vi "ai_oneshot_ext_trig_in.vi"() -> ()   [LabVIEW 2020]
uses:
  <vilib>/Platform/TimedLoop/XDataNode/timing_clust.ctl
  <vilib>/Platform/TimedLoop/XDataNode/nitl_modes.ctl
  <vilib>/Platform/TimedLoop/XDataNode/wakeup.ctl
  <vilib>/platform/TimedLoop/XDataNode/XDataNode.xnode
  <vilib>/Platform/TimedLoop/XDataNode/XDNodeRunTimeDep.lvlib
panel:
  out "loop":i32
  in  "stop":bool
  in  "AiOneShotPoints":u32=500
  out "error out":errorcluster caption="错误输出"
  out "AiFifoResidual":i32
  out "波形图":sgl[][](graph)=[[1.0535451, 1.0535451, 1.0633912, 1.0584682, 1.0535451, 1.0535451, 1.0535451, 1.0535451, 1.0535451, 1.0535451, 1.0535451, 1.0486219, 1.0535451, 1.0486219, 1.0535451, 1.0535451, 1.0535451, 1.0535451, 1.0535451, 1.0535451, 1.0535451, 1.0535451, 1.0486219, 1.0535451, 1.0535451, 1.0535451, 1.0535451, 1.0535451, 1.0535451, 1.0535451, 1.0535451, 1.0486219, 1.0535451, 1.0535451, 1.0535451, 1.0535451, 1.0535451, 1.0535451, 1.0535451, 1.0584682, 1.0535451, 1.0535451, 1.0535451, 1.0535451, 1.0535451, 1.0535451, 1.0535451, 1.0535451, 1.0584682, 1.0535451, 1.0535451, 1.0535451, 1.0535451, 1.0535451, 1.0535451, 1.0535451, 1.0584682, 1.0584682, 1.0535451, 1.0584682, 1.0584682, 1.0584682, 1.0535451, 1.0535451, 1.0584682, 1.0535451, 1.0584682, 1.0535451, 1.0535451, 1.0535451, 1.0584682, 1.0535451, 1.0535451, 1.0535451, 1.0535451, 1.0584682, 1.0535451, 1.0535451, 1.0584682, 1.0535451, 1.0535451, 1.0535451, 1.0535451, 1.0535451, 1.0584682, 1.0535451, 1.0535451, 1.0535451, 1.0535451, 1.0535451, 1.0535451, 1.0535451, 1.0535451, 1.0535451, 1.0535451, 1.0535451, 1.0535451, 1.0535451, 1.0535451, 1.0535451, 1.0535451, 1.0535451, 1.0535451, 1.0486219, 1.0535451, 1.0535451, 1.0535451, 1.0535451, 1.0535451, 1.0535451, 1.0535451, 1.0535451, 1.0535451, 1.0535451, 1.0535451, 1.0535451, 1.0535451, 1.0535451, 1.0535451, 1.0535451, 1.0535451, 1.0535451, 1.0535451, 1.0535451, 1.0535451, 1.0535451, 1.0535451, 1.0535451, 1.0535451, 1.0535451, 1.0535451, 1.0535451, 1.0535451, 1.0584682, 1.0584682, 1.0584682, 1.0535451, 1.0584682, 1.0584682, 1.0584682, 1.0584682, 1.0633912, 1.0633912, 1.0633912, 1.0633912, 1.0633912, 1.0633912, 1.0633912, 1.0584682, 1.0633912, 1.0584682, 1.0584682, 1.0584682, 1.0584682, 1.0584682, 1.0584682, 1.0633912, 1.0584682, 1.0584682, 1.0584682, 1.0633912, 1.0633912, 1.0584682, 1.0584682, 1.0584682, 1.0633912, 1.0584682, 1.0584682, 1.0584682, 1.0584682, 1.0584682, 1.0584682, 1.0584682, 1.0584682, 1.0584682, 1.0535451, 1.0535451, 1.0535451, 1.0535451, 1.0535451, 1.0535451, 1.0535451, 1.0535451, 1.0535451, 1.0486219, 1.0535451, 1.0535451, 1.0535451, 1.0535451, 1.0535451, 1.0535451, 1.0535451, 1.0535451, 1.0535451, 1.0535451, 1.0535451, 1.0535451, 1.0535451, 1.0535451, 1.0535451, 1.0535451, 1.0535451, 1.0535451, 1.0535451, 1.0535451, 1.0535451, 1.0535451, 1.0535451, 1.0535451, 1.0535451, 1.0584682, 1.0535451, 1.0535451, 1.0584682, 1.0584682, 1.0584682, 1.0584682, 1.0584682, 1.0584682, 1.0584682, 1.0535451, 1.0584682, 1.0584682, 1.0584682, 1.0584682, 1.0584682, 1.0584682, 1.0584682, 1.0584682, 1.0535451, 1.0584682, 1.0584682, 1.0584682, 1.0584682, 1.0584682, 1.0584682, 1.0584682, 1.0633912, 1.0584682, 1.0584682, 1.0584682, 1.0584682, 1.0584682, 1.0584682, 1.0584682, 1.0584682, 1.0584682, 1.0535451, 1.0535451, 1.0584682, 1.0584682, 1.0535451, 1.0535451, 1.0535451, 1.0535451, 1.0535451, 1.0486219, 1.0535451, 1.0535451, 1.0535451, 1.0535451, 1.0535451, 1.0535451, 1.0535451, 1.0535451, 1.0486219, 1.0535451, 1.0535451, 1.0535451, 1.0486219, 1.0486219, 1.0486219, 1.0486219, 1.0486219, 1.0486219, 1.0486219, 1.0486219, 1.0486219, 1.0486219, 1.0486219, 1.0486219, 1.0486219, 1.0486219, 1.0486219, 1.0486219, 1.0486219, 1.0486219, 1.0486219, 1.0486219, 1.0486219, 1.0486219, 1.0535451, 1.0486219, 1.0486219, 1.0486219, 1.0486219, 1.0486219, 1.0486219, 1.0486219, 1.0486219, 1.0486219, 1.0486219, 1.0486219, 1.0486219, 1.0535451, 1.0486219, 1.0486219, 1.0535451, 1.0535451, 1.0535451, 1.0486219, 1.0535451, 1.0535451, 1.0535451, 1.0535451, 1.0535451, 1.0535451, 1.0584682, 1.0584682, 1.0584682, 1.0584682, 1.0584682, 1.0633912, 1.0633912, 1.0584682, 1.0633912, 1.0633912, 1.0633912, 1.0633912, 1.0633912, 1.0633912, 1.0633912, 1.0633912, 1.0633912, 1.0633912, 1.0683143, 1.0683143, 1.0633912, 1.0633912, 1.0633912, 1.0683143, 1.0633912, 1.0683143, 1.0683143, 1.0683143, 1.0683143, 1.0633912, 1.0683143, 1.0683143, 1.0683143, 1.0683143, 1.0683143, 1.0683143, 1.0633912, 1.0683143, 1.0633912, 1.0633912, 1.0633912, 1.0633912, 1.0633912, 1.0633912, 1.0633912, 1.0633912, 1.0633912, 1.0584682, 1.0633912, 1.0584682, 1.0584682, 1.0584682, 1.0584682, 1.0584682, 1.0584682, 1.0584682, 1.0535451, 1.0584682, 1.0584682, 1.0584682, 1.0584682, 1.0584682, 1.0584682, 1.0535451, 1.0535451, 1.0486219, 1.0535451, 1.0535451, 1.0535451, 1.0535451, 1.0535451, 1.0486219, 1.0486219, 1.0486219, 1.0486219, 1.0486219, 1.0486219, 1.0486219, 1.0486219, 1.0486219, 1.0486219, 1.0486219, 1.0486219, 1.0436989, 1.0486219, 1.0486219, 1.0486219, 1.0486219, 1.0486219, 1.0486219, 1.0486219, 1.0486219, 1.0436989, 1.0486219, 1.0486219, 1.0486219, 1.0486219, 1.0486219, 1.0486219, 1.0486219, 1.0486219, 1.0436989, 1.0486219, 1.0535451, 1.0486219, 1.0486219, 1.0535451, 1.0486219, 1.0535451, 1.0535451, 1.0486219, 1.0535451, 1.0535451, 1.0535451, 1.0535451, 1.0535451, 1.0535451, 1.0535451, 1.0535451, 1.0486219, 1.0535451, 1.0535451, 1.0535451, 1.0535451, 1.0535451, 1.0535451, 1.0535451, 1.0535451, 1.0486219, 1.0535451, 1.0535451, 1.0535451, 1.0535451, 1.0535451, 1.0535451, 1.0535451, 1.0535451, 1.0535451, 1.0535451, 1.0535451, 1.0535451, 1.0535451, 1.0535451, 1.0535451, 1.0535451, 1.0584682, 1.0535451, 1.0584682, 1.0584682, 1.0584682, 1.0584682, 1.0584682, 1.0584682, 1.0584682, 1.0584682, 1.0584682, 1.0633912, 1.0633912, 1.0633912, 1.0633912, 1.0633912, 1.0633912, 1.0633912, 1.0633912, 1.0584682, 1.0633912, 1.0633912, 1.0633912, 1.0633912, 1.0633912, 1.0633912, 1.0633912, 1.0633912, 1.0633912, 1.0633912, 1.0633912, 1.0683143, 1.0633912, 1.0633912, 1.0683143, 1.0633912, 1.0683143, 1.0633912, 1.0633912, 1.0683143, 1.0683143, 1.0633912, 1.0633912, 1.0633912, 1.0633912, 1.0584682, 1.0535451, 1.0486219, 1.0436989, 1.0436989, 1.0387758, 1.0338527, 1.0338527, 1.0338527, 1.0338527, 1.0240065, 1.0289296, 1.0289296, 1.0289296, 1.0289296, 1.0289296, 1.0289296, 1.0289296, 1.0289296, 1.0240065, 1.0338527, 1.0338527, 1.0338527, 1.0338527, 1.0338527, 1.0387758, 1.0387758, 1.0387758, 1.0387758, 1.0436989, 1.0436989, 1.0436989, 1.0436989, 1.0486219, 1.0486219, 1.0486219, 1.0535451, 1.0535451, 1.0535451, 1.0535451, 1.0584682, 1.0584682, 1.0584682], [1.0581981, 1.0581981, 1.0581981, 1.0631206, 1.0581981, 1.0581981, 1.0581981, 1.0581981, 1.0581981, 1.0581981, 1.0581981, 1.0532755, 1.0581981, 1.0581981, 1.0581981, 1.0581981, 1.0581981, 1.0581981, 1.0581981, 1.0631206, 1.0581981, 1.0631206, 1.0631206, 1.0631206, 1.0631206, 1.0631206, 1.0631206, 1.0680432, 1.0631206, 1.0631206, 1.0680432, 1.0631206, 1.0680432, 1.0631206, 1.0631206, 1.0631206, 1.0631206, 1.0631206, 1.0581981, 1.0631206, 1.0631206, 1.0631206, 1.0581981, 1.0581981, 1.0581981, 1.0581981, 1.0581981, 1.0581981, 1.0581981, 1.0581981, 1.0581981, 1.0532755, 1.0532755, 1.0532755, 1.0532755, 1.0532755, 1.0483528, 1.0532755, 1.0532755, 1.0532755, 1.0532755, 1.0532755, 1.0483528, 1.0532755, 1.0483528, 1.0434302, 1.0483528, 1.0483528, 1.0483528, 1.0483528, 1.0483528, 1.0483528, 1.0483528, 1.0483528, 1.0434302, 1.0483528, 1.0434302, 1.0483528, 1.0434302, 1.0434302, 1.0434302, 1.0434302, 1.0483528, 1.0434302, 1.0483528, 1.0483528, 1.0483528, 1.0434302, 1.0483528, 1.0483528, 1.0483528, 1.0483528, 1.0434302, 1.0483528, 1.0483528, 1.0532755, 1.0483528, 1.0483528, 1.0483528, 1.0483528, 1.0483528, 1.0483528, 1.0532755, 1.0532755, 1.0532755, 1.0532755, 1.0532755, 1.0532755, 1.0532755, 1.0532755, 1.0532755, 1.0581981, 1.0581981, 1.0581981, 1.0581981, 1.0581981, 1.0581981, 1.0631206, 1.0631206, 1.0581981, 1.0631206, 1.0631206, 1.0631206, 1.0631206, 1.0680432, 1.0680432, 1.0680432, 1.0680432, 1.0631206, 1.0680432, 1.0631206, 1.0631206, 1.0631206, 1.0631206, 1.0631206, 1.0631206, 1.0581981, 1.0581981, 1.0631206, 1.0581981, 1.0631206, 1.0581981, 1.0581981, 1.0581981, 1.0581981, 1.0581981, 1.0532755, 1.0581981, 1.0532755, 1.0581981, 1.0532755, 1.0532755, 1.0532755, 1.0532755, 1.0532755, 1.0483528, 1.0483528, 1.0483528, 1.0483528, 1.0483528, 1.0483528, 1.0483528, 1.0483528, 1.0483528, 1.0434302, 1.0483528, 1.0483528, 1.0483528, 1.0483528, 1.0483528, 1.0483528, 1.0483528, 1.0483528, 1.0434302, 1.0483528, 1.0483528, 1.0483528, 1.0483528, 1.0532755, 1.0532755, 1.0532755, 1.0532755, 1.0532755, 1.0532755, 1.0532755, 1.0532755, 1.0532755, 1.0532755, 1.0581981, 1.0581981, 1.0581981, 1.0532755, 1.0532755, 1.0532755, 1.0532755, 1.0532755, 1.0532755, 1.0532755, 1.0532755, 1.0532755, 1.0532755, 1.0532755, 1.0581981, 1.0581981, 1.0532755, 1.0581981, 1.0581981, 1.0581981, 1.0581981, 1.0532755, 1.0581981, 1.0581981, 1.0581981, 1.0532755, 1.0581981, 1.0581981, 1.0581981, 1.0581981, 1.0532755, 1.0581981, 1.0581981, 1.0581981, 1.0532755, 1.0581981, 1.0532755, 1.0532755, 1.0532755, 1.0532755, 1.0532755, 1.0532755, 1.0532755, 1.0532755, 1.0532755, 1.0532755, 1.0532755, 1.0532755, 1.0483528, 1.0532755, 1.0532755, 1.0532755, 1.0532755, 1.0532755, 1.0532755, 1.0532755, 1.0532755, 1.0483528, 1.0532755, 1.0532755, 1.0483528, 1.0483528, 1.0532755, 1.0532755, 1.0483528, 1.0483528, 1.0483528, 1.0483528, 1.0483528, 1.0483528, 1.0483528, 1.0483528, 1.0483528, 1.0532755, 1.0532755, 1.0483528, 1.0532755, 1.0532755, 1.0532755, 1.0532755, 1.0532755, 1.0532755, 1.0532755, 1.0532755, 1.0483528, 1.0532755, 1.0532755, 1.0532755, 1.0532755, 1.0532755, 1.0532755, 1.0532755, 1.0532755, 1.0483528, 1.0532755, 1.0532755, 1.0581981, 1.0532755, 1.0581981, 1.0581981, 1.0581981, 1.0581981, 1.0532755, 1.0581981, 1.0581981, 1.0581981, 1.0581981, 1.0581981, 1.0581981, 1.0581981, 1.0581981, 1.0581981, 1.0631206, 1.0631206, 1.0631206, 1.0631206, 1.0631206, 1.0631206, 1.0631206, 1.0631206, 1.0631206, 1.0680432, 1.0680432, 1.0680432, 1.0680432, 1.0680432, 1.0680432, 1.0680432, 1.0680432, 1.0631206, 1.0680432, 1.0631206, 1.0631206, 1.0631206, 1.0631206, 1.0631206, 1.0631206, 1.0631206, 1.0581981, 1.0631206, 1.0631206, 1.0631206, 1.0581981, 1.0581981, 1.0581981, 1.0581981, 1.0581981, 1.0532755, 1.0581981, 1.0532755, 1.0532755, 1.0532755, 1.0532755, 1.0532755, 1.0532755, 1.0532755, 1.0483528, 1.0483528, 1.0483528, 1.0532755, 1.0483528, 1.0483528, 1.0483528, 1.0483528, 1.0483528, 1.0434302, 1.0483528, 1.0483528, 1.0483528, 1.0434302, 1.0434302, 1.0434302, 1.0434302, 1.0483528, 1.0434302, 1.0483528, 1.0483528, 1.0483528, 1.0434302, 1.0434302, 1.0434302, 1.0434302, 1.0434302, 1.0434302, 1.0434302, 1.0434302, 1.0483528, 1.0434302, 1.0483528, 1.0483528, 1.0483528, 1.0483528, 1.0434302, 1.0483528, 1.0483528, 1.0483528, 1.0483528, 1.0483528, 1.0483528, 1.0532755, 1.0483528, 1.0483528, 1.0483528, 1.0532755, 1.0532755, 1.0483528, 1.0532755, 1.0532755, 1.0532755, 1.0532755, 1.0483528, 1.0532755, 1.0532755, 1.0532755, 1.0532755, 1.0532755, 1.0532755, 1.0581981, 1.0581981, 1.0532755, 1.0581981, 1.0581981, 1.0581981, 1.0532755, 1.0581981, 1.0581981, 1.0581981, 1.0581981, 1.0532755, 1.0581981, 1.0581981, 1.0581981, 1.0581981, 1.0581981, 1.0581981, 1.0581981, 1.0581981, 1.0532755, 1.0581981, 1.0581981, 1.0581981, 1.0532755, 1.0581981, 1.0581981, 1.0581981, 1.0581981, 1.0532755, 1.0581981, 1.0581981, 1.0581981, 1.0532755, 1.0581981, 1.0581981, 1.0581981, 1.0581981, 1.0532755, 1.0581981, 1.0581981, 1.0581981, 1.0581981, 1.0581981, 1.0581981, 1.0581981, 1.0581981, 1.0581981, 1.0581981, 1.0581981, 1.0631206, 1.0581981, 1.0581981, 1.0631206, 1.0631206, 1.0631206, 1.0581981, 1.0631206, 1.0631206, 1.0631206, 1.0631206, 1.0631206, 1.0631206, 1.0631206, 1.0631206, 1.0581981, 1.0631206, 1.0631206, 1.0631206, 1.0631206, 1.0631206, 1.0631206, 1.0631206, 1.0631206, 1.0581981, 1.0581981, 1.0581981, 1.0581981, 1.0581981, 1.0581981, 1.0532755, 1.0532755, 1.0532755, 1.0483528, 1.0532755, 1.0532755, 1.0532755, 1.0483528, 1.0532755, 1.0532755, 1.0483528, 1.0483528, 1.0434302, 1.0483528, 1.0483528, 1.0483528, 1.0483528, 1.0483528, 1.0483528, 1.0434302, 1.0434302, 1.0434302, 1.0434302, 1.0237398, 1.0040494, 0.9695912, 0.94005567, 0.9055974, 0.8760618, 0.8465262, 0.8268358, 0.8022228, 0.78745496, 0.77760977, 0.77268714, 0.76776457, 0.76776457, 0.77760977, 0.78745496, 0.8022228, 0.812068, 0.8317584, 0.8514488, 0.8760618, 0.8957522, 0.9203652, 0.94497824, 0.9695912, 0.9942042, 1.0188173, 1.0434302, 1.0680432, 1.0877336, 1.107424, 1.1271144, 1.1468048, 1.1664952, 1.1763405, 1.1960309, 1.2107987, 1.2206439, 1.230489, 1.2452569, 1.2551022, 1.2600247], [1.1697962, 1.1697962, 1.1747131, 1.1697962, 1.1697962, 1.1697962, 1.1697962, 1.1697962, 1.1697962, 1.1697962, 1.1747131, 1.1747131, 1.1747131, 1.1747131, 1.1747131, 1.1796299, 1.1796299, 1.1796299, 1.1845467, 1.1845467, 1.1845467, 1.1845467, 1.1845467, 1.1894635, 1.1894635, 1.1894635, 1.1943805, 1.1943805, 1.1943805, 1.1943805, 1.1943805, 1.1992973, 1.1992973, 1.1992973, 1.2042141, 1.2042141, 1.2042141, 1.2042141, 1.209131, 1.209131, 1.209131, 1.209131, 1.2140479, 1.2140479, 1.2140479, 1.2140479, 1.2189647, 1.2189647, 1.2189647, 1.2189647, 1.2189647, 1.2238815, 1.2238815, 1.2238815, 1.2238815, 1.2287983, 1.2287983, 1.2287983, 1.2337153, 1.2337153, 1.2337153, 1.2337153, 1.2337153, 1.2386321, 1.2386321, 1.2386321, 1.2386321, 1.2435489, 1.2435489, 1.2435489, 1.2435489, 1.2435489, 1.2484658, 1.2484658, 1.2484658, 1.2533826, 1.2533826, 1.2533826, 1.2533826, 1.2533826, 1.2582995, 1.2582995, 1.2582995, 1.2632163, 1.2632163, 1.2632163, 1.2632163, 1.268133, 1.268133, 1.268133, 1.268133, 1.27305, 1.27305, 1.27305, 1.27305, 1.2779669, 1.2779669, 1.2779669, 1.2779669, 1.2779669, 1.2828836, 1.2828836, 1.2828836, 1.2828836, 1.2878006, 1.2878006, 1.2878006, 1.2878006, 1.2927173, 1.2927173, 1.2927173, 1.2927173, 1.2976342, 1.2976342, 1.2976342, 1.2976342, 1.302551, 1.302551, 1.302551, 1.302551, 1.3074678, 1.3074678, 1.3074678, 1.3074678, 1.3123847, 1.3123847, 1.3123847, 1.3123847, 1.3173016, 1.3173016, 1.3173016, 1.3173016, 1.3222184, 1.3222184, 1.3222184, 1.3222184, 1.3222184, 1.3271353, 1.3271353, 1.3271353, 1.3271353, 1.3320521, 1.3320521, 1.3320521, 1.336969, 1.336969, 1.336969, 1.336969, 1.3418858, 1.3418858, 1.3418858, 1.3418858, 1.3418858, 1.3468026, 1.3468026, 1.3468026, 1.3517195, 1.3517195, 1.3517195, 1.3517195, 1.3517195, 1.3566363, 1.3566363, 1.3566363, 1.3566363, 1.3615532, 1.3615532, 1.3615532, 1.3615532, 1.3664701, 1.3664701, 1.3664701, 1.3664701, 1.3713869, 1.3713869, 1.3713869, 1.3713869, 1.3763037, 1.3763037, 1.3763037, 1.3763037, 1.3812206, 1.3812206, 1.3812206, 1.3812206, 1.3861374, 1.3861374, 1.3861374, 1.3861374, 1.3861374, 1.3910543, 1.3910543, 1.3910543, 1.3910543, 1.3959711, 1.3959711, 1.3959711, 1.3959711, 1.400888, 1.400888, 1.400888, 1.4058049, 1.4058049, 1.4058049, 1.4058049, 1.4058049, 1.4107217, 1.4107217, 1.4107217, 1.4156384, 1.4156384, 1.4156384, 1.4156384, 1.4205554, 1.4205554, 1.4205554, 1.4205554, 1.4205554, 1.4254721, 1.4254721, 1.4254721, 1.4254721, 1.430389, 1.430389, 1.430389, 1.430389, 1.4353058, 1.4353058, 1.4353058, 1.4353058, 1.4402226, 1.4402226, 1.4402226, 1.4451396, 1.4451396, 1.4451396, 1.4451396, 1.4451396, 1.4500564, 1.4500564, 1.4500564, 1.4500564, 1.4549732, 1.4549732, 1.4549732, 1.4549732, 1.45989, 1.45989, 1.45989, 1.45989, 1.4648069, 1.4648069, 1.4648069, 1.4648069, 1.4697238, 1.4697238, 1.4697238, 1.4697238, 1.4697238, 1.4746406, 1.4746406, 1.4746406, 1.4795574, 1.4795574, 1.4795574, 1.4795574, 1.4844744, 1.4844744, 1.4844744, 1.4844744, 1.4893912, 1.4893912, 1.4893912, 1.4893912, 1.4893912, 1.494308, 1.494308, 1.494308, 1.494308, 1.4992248, 1.4992248, 1.4992248, 1.5041417, 1.5041417, 1.5041417, 1.5041417, 1.5090586, 1.5090586, 1.5090586, 1.5090586, 1.5090586, 1.5139754, 1.5139754, 1.5139754, 1.5139754, 1.5188922, 1.5188922, 1.5188922, 1.5188922, 1.5238092, 1.5238092, 1.5238092, 1.5238092, 1.528726, 1.528726, 1.528726, 1.528726, 1.5336428, 1.5336428, 1.5336428, 1.5336428, 1.5385596, 1.5385596, 1.5385596, 1.5385596, 1.5434763, 1.5434763, 1.5434763, 1.5434763, 1.5483934, 1.5483934, 1.5483934, 1.5483934, 1.5483934, 1.5533102, 1.5533102, 1.5533102, 1.5533102, 1.558227, 1.558227, 1.558227, 1.5631438, 1.5631438, 1.5631438, 1.5631438, 1.5631438, 1.5680608, 1.5680608, 1.5680608, 1.5680608, 1.5729775, 1.5729775, 1.5729775, 1.5729775, 1.5778943, 1.5778943, 1.5778943, 1.5778943, 1.5828111, 1.5828111, 1.5828111, 1.5828111, 1.5877281, 1.5877281, 1.5877281, 1.5877281, 1.5926449, 1.5926449, 1.5926449, 1.5926449, 1.5975617, 1.5975617, 1.5975617, 1.6024786, 1.6024786, 1.6024786, 1.6024786, 1.6073955, 1.6073955, 1.6073955, 1.6073955, 1.6073955, 1.6123123, 1.6123123, 1.6123123, 1.6123123, 1.6172291, 1.6172291, 1.6172291, 1.6172291, 1.6221459, 1.6221459, 1.6221459, 1.6221459, 1.6221459, 1.6270629, 1.6270629, 1.6270629, 1.6319797, 1.6319797, 1.6319797, 1.6319797, 1.6368965, 1.6368965, 1.6368965, 1.6368965, 1.6418134, 1.6418134, 1.6418134, 1.6418134, 1.6467302, 1.6467302, 1.6467302, 1.6467302, 1.6467302, 1.6516471, 1.6516471, 1.6516471, 1.6516471, 1.6565639, 1.6565639, 1.6565639, 1.6565639, 1.6614807, 1.6614807, 1.6614807, 1.6663976, 1.6663976, 1.6663976, 1.6663976, 1.6663976, 1.6713145, 1.6713145, 1.6713145, 1.6762313, 1.6762313, 1.6762313, 1.6762313, 1.6762313, 1.6762313, 1.6811482, 1.6811482, 1.6811482, 1.686065, 1.686065, 1.686065, 1.686065, 1.686065, 1.6909819, 1.6909819, 1.6909819, 1.6958987, 1.6958987, 1.6958987, 1.6958987, 1.6958987, 1.7008154, 1.7008154, 1.7008154, 1.7008154, 1.7057323, 1.7057323, 1.7057323, 1.7106493, 1.7106493, 1.7106493, 1.7106493, 1.7106493, 1.715566, 1.715566, 1.715566, 1.715566, 1.720483, 1.720483, 1.720483, 1.7253997, 1.7253997, 1.7253997, 1.7253997, 1.7303165, 1.7303165, 1.7303165, 1.7303165, 1.7303165, 1.7352334, 1.7352334, 1.7352334, 1.7352334, 1.7401502, 1.7401502, 1.7401502, 1.7401502, 1.7450671, 1.7450671, 1.7450671, 1.7450671, 1.7499839, 1.7499839, 1.7499839, 1.7499839, 1.7549008, 1.7549008, 1.7549008, 1.7549008, 1.7598177, 1.7598177, 1.7598177, 1.7598177, 1.7647345, 1.7647345, 1.7647345, 1.7598177, 1.7647345, 1.7696513, 1.7696513, 1.6663976, 1.3271353, 1.2189647, 1.1845467, 1.1747131, 1.1697962, 1.1697962, 1.1697962, 1.1697962, 1.1697962, 1.1697962, 1.1697962, 1.1697962, 1.1697962, 1.1697962, 1.1697962, 1.1697962, 1.1697962, 1.1697962, 1.1697962, 1.1697962, 1.1697962, 1.1697962, 1.1697962, 1.1697962, 1.1697962, 1.1697962, 1.1697962, 1.1697962, 1.1697962, 1.1697962, 1.1697962, 1.1697962, 1.1697962, 1.1697962, 1.1697962, 1.1697962, 1.1697962, 1.1697962, 1.1697962, 1.1697962, 1.1697962, 1.1697962, 1.1697962, 1.1697962]]
  in  "SamplePeriod(ns)":u32=2000
  in  "ChanSel":bool[](array[boolean])=[TRUE, TRUE, TRUE, FALSE, FALSE, FALSE, FALSE, FALSE, FALSE, FALSE, FALSE, FALSE, FALSE, FALSE, FALSE, FALSE, FALSE, FALSE, FALSE, FALSE, FALSE, FALSE, FALSE, FALSE]
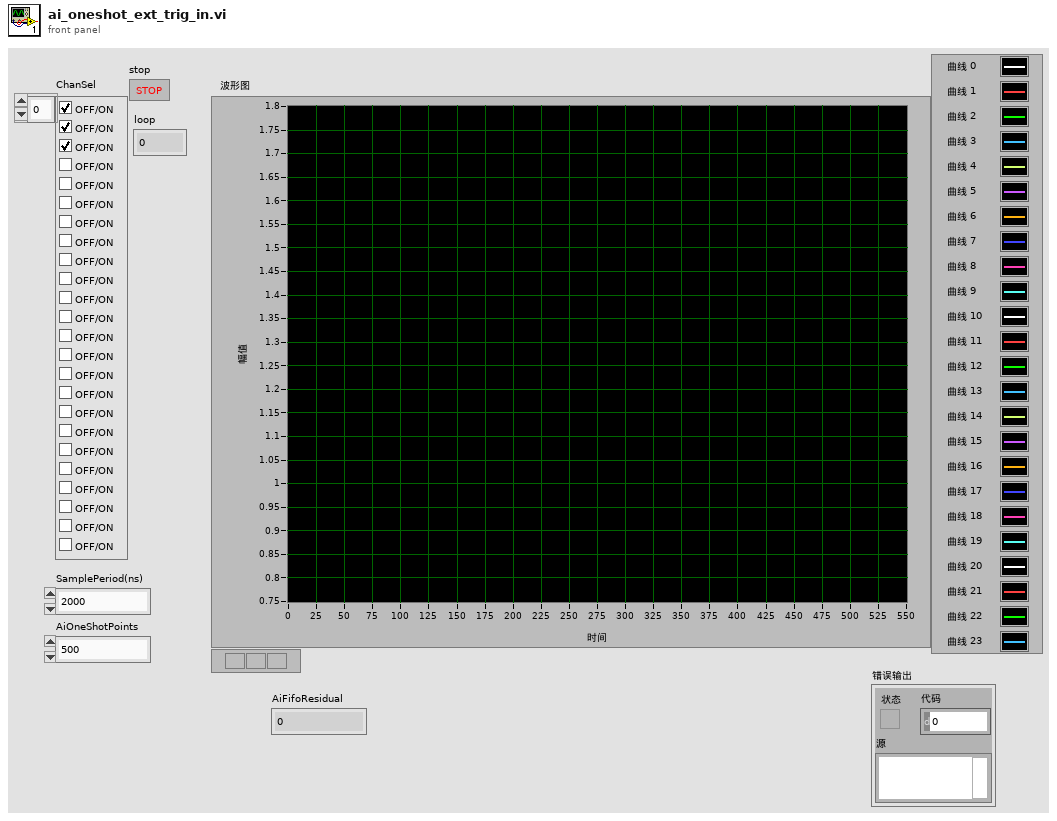
[diagram p1: front panel]
types:
  T1 = typedef "XDNodeRunTimeDep.lvlib/timing_clust.ctl" = cluster{"Expected End [f-1]":u64, "Actual End [f-1]":u64, "Finished Late? [f-1]":bool, "Expected End [i-1]":u64, "Actual End [i-1]":u64, "Finished Late? [i-1]":bool, "Expected Start [i]":u64, "Actual Start [i]":u64, "Expected Start [f]":u64, "Actual Start [f]":u64, "Source Name":string, "Structure Name":string, "Period":i64, "Deadline":i64, "Offset":i64, "Start":i64, "Priority":i32, "Timeout":i32, "Mode":T2, "Wakeup Reason":T3, "Error":errorcluster, "Source Type":string, "Secondary Source Type":string, "Global End Time":u64, "Global Start Time":u64, "Frame Duration":u64, "Iteration Duration":u64, "Assigned CPU":i32, "I/O Scan Engine Mode":u32}
  T2 = typedef "XDNodeRunTimeDep.lvlib/nitl_modes.ctl" = enum32{"No Change", "Process missed periods, maintain original phase", "Discard missed periods, maintain original phase", "Process missed periods, ignore original phase", "Discard missed periods, ignore original phase"}
  T3 = typedef "XDNodeRunTimeDep.lvlib/wakeup.ctl" = enum32{"Normal", "Aborted", "Asynchronous wakeup", "Timing source error", "Timed loop error", "Timeout"}
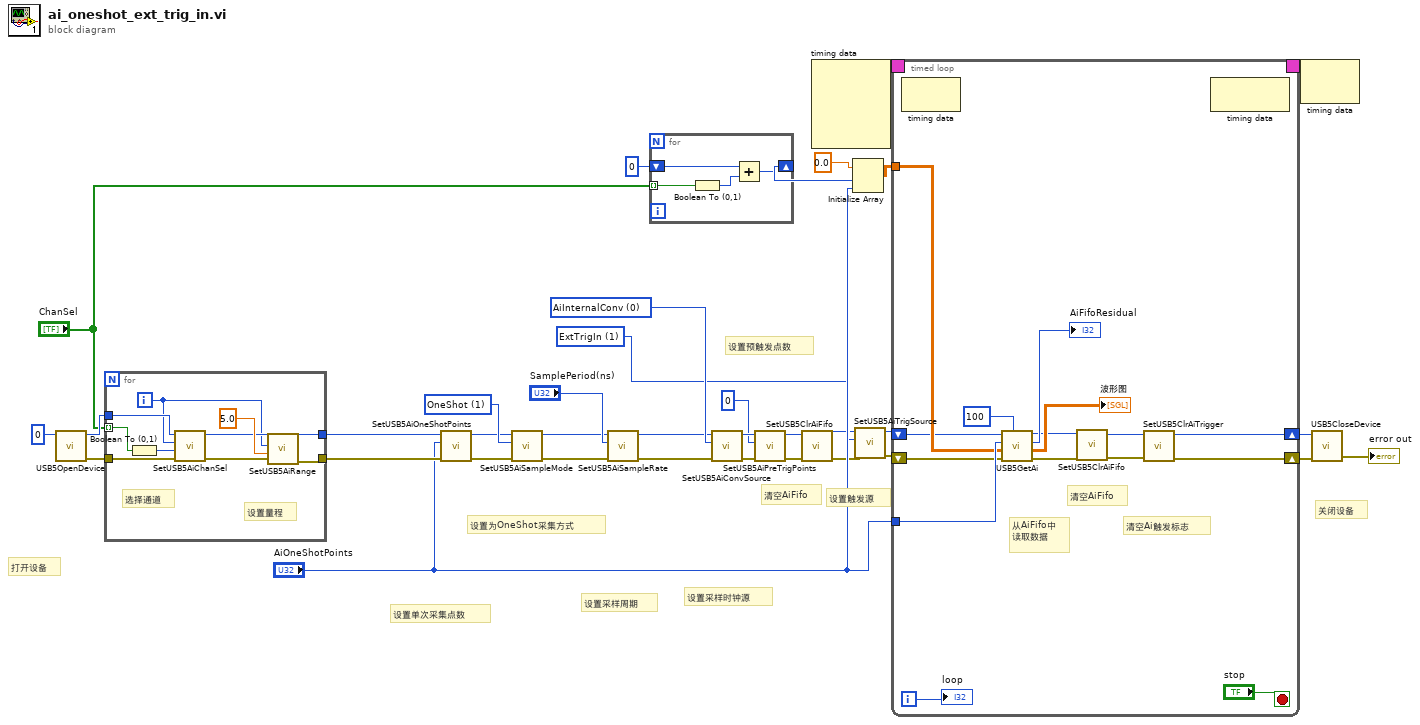
[diagram p0: block diagram]
diagram:
  w12 = u8 0 items=["AiInternalConv"=0, "ConvIn"=1, "DiConv"=3, "DoConv"=4, "Ao0Conv"=5, "Ao1Conv"=6, "Ao2Conv"=7, "Ao3Conv"=8] ("AiConvSource")
  w9 = u8 1 items=["AiSoftTrig"=0, "ExtTrigIn"=1, "Din0RisingEdge"=2, "Din1RisingEdge"=3, "Din2RisingEdge"=4, "Din3RisingEdge"=5, "WithDiTrig"=7, "WithDoTrig"=8, "WithAo0Trig"=9, "WithAo1Trig"=10, "WithAo2Trig"=11, "WithAo3Trig"=12, "GlobalSoftTrig"=255] ("AiTrigSource")
  w32 = u8 1 items=["Continuous", "OneShot"] ("AiSampleMode")
  # "关闭设备"
  # "清空AiFifo"
  # "设置预触发点数"
  # "设置采样时钟源"
  # "设置触发源"
  # "设置采样周期"
  # "设置为OneShot采集方式"
  # "设置单次采集点数"
  # "打开设备"
  n1 = call "USB5OpenDevice.vi"("DevIndex"=0) -> ("error out"=w33:errorcluster, "DevIndex Out"=w34:i32)  [unwired: 9 in]
  n2 = for {
    tunnel: w34 -> [w45]
    tunnel: w33 -> [w44]
    tunnel: [w37] -> w14
    tunnel: [w36] -> w13
    tunnel: "ChanSel" -> [w42] mode=indexing
    i -> [w39]
    # "设置量程"
    # "选择通道"
    n3 = Boolean To (0,1)(Boolean=w42) -> (0, 1=w43:i16)
    n4 = call "SetUSB5AiChanSel.vi"("错误输入（无错误）"=w44, "Sel"=w43, "Chan"=w39, "DevIndex"=w45) -> ("错误输出"=w38:errorcluster, "DevIndex Out"=w40:i32)  [unwired: 6 in]
    n5 = call "SetUSB5AiRange.vi"("错误输入（无错误）"=w38, "AiRange"=sgl 5.0, "Chan"=w39, "DevIndex"=w40) -> ("错误输出"=w36:errorcluster, "DevIndex Out"=w37:i32)  [unwired: 6 in]
  }
  n6 = call "SetUSB5AiOneShotPoints.vi"("错误输入（无错误）"=w13, "AiOneShotPoints"="AiOneShotPoints", "DevIndex"=w14) -> ("错误输出"=w23:errorcluster, "DevIndex Out"=w24:i32)  [unwired: 7 in]
  n7 = call "SetUSB5AiSampleMode.vi"("错误输入（无错误）"=w23, "AiSampleMode"=w32, "DevIndex"=w24) -> ("错误输出"=w15:errorcluster, "DevIndex Out"=w16:i32)  [unwired: 7 in]
  n8 = call "SetUSB5AiSampleRate.vi"("错误输入（无错误）"=w15, "SamplePeriod(ns)"="SamplePeriod(ns)", "DevIndex"=w16) -> ("错误输出"=w5:errorcluster, "DevIndex Out"=w6:i32)  [unwired: 7 in]
  n9 = for {
    tunnel: "ChanSel" -> [w49] mode=indexing
    shift-right: [w46] -> w25
    shift-left: i16 0 -> [w47]
    n10 = Boolean To (0,1)(Boolean=w49) -> (0, 1=w48:i16)
    n11 = Add(x=w47, y=w48) -> (x+y=w46:i16)
  }
  n12 = call "SetUSB5AiConvSource.vi"("错误输入（无错误）"=w5, "AiConvSource"=w12, "DevIndex"=w6) -> ("错误输出"=w21:errorcluster, "DevIndex Out"=w20:i32)  [unwired: 7 in]
  n13 = call "SetUSB5AiPreTrigPoints.vi"("错误输入（无错误）"=w21, "AiPreTrigPoints"=u32 0, "DevIndex"=w20) -> ("错误输出"=w18:errorcluster, "DevIndex Out"=w19:i32)  [unwired: 7 in]
  n14 = call "SetUSB5ClrAiFifo.vi"("错误输入（无错误）"=w18, "DevIndex"=w19) -> ("错误输出"=w4:errorcluster, "DevIndex Out"=w8:i32)  [unwired: 8 in]
  n15 = node-c288() -> (w2:T1)  [unwired: 4 in]
  n16 = Initialize Array(sgl 0.0 ("元素"), w25, "AiOneShotPoints") -> (w17:sgl[][])
  n17 = call "SetUSB5AiTrigSource.vi"("错误输入（无错误）"=w4, "AiTrigSource"=w9, "DevIndex"=w8) -> ("错误输出"=w3:errorcluster, "DevIndex Out"=w7:i32)  [unwired: 7 in]
  n18 = timed-loop {
    tunnel: "AiOneShotPoints" -> [w62]
    tunnel: w17 -> [w61]
    shift-right: [w54] -> w28
    shift-left: w3 -> [w57]
    shift-right: [w55] -> w27
    shift-left: w7 -> [w58]
    timing: w2 -> [_]
    timing-out: [_] -> w1
    i -> [w56]
    stop <- "stop" stop-if-true
    # "清空AiFifo"
    # "清空Ai触发标志"
    # "从AiFifo中\n读取数据"
    n19 = node-c288() -> ()  [unwired: 1 in, 1 out]
    n20 = call "USB5GetAi.vi"("TimeOut"=100, "错误输入（无错误）"=w57, "Ai"=w61, "Points"=w62, "DevIndex"=w58) -> ("错误输出"=w53:errorcluster, "Ai Out"=→"波形图":sgl[][], "AiFifoUsed"=→"AiFifoResidual":i32, "DevIndex Out"=w50:i32)  [unwired: 3 in]
    n21 = call "SetUSB5ClrAiFifo.vi"("错误输入（无错误）"=w53, "DevIndex"=w50) -> ("错误输出"=w52:errorcluster, "DevIndex Out"=w51:i32)  [unwired: 8 in]
    n22 = call "SetUSB5ClrAiTrigger.vi"("错误输入（无错误）"=w52, "DevIndex"=w51) -> ("错误输出"=w54:errorcluster, "DevIndex Out"=w55:i32)  [unwired: 8 in]
    n23 = node-c288() -> ()  [unwired: 1 in, 1 out]
    "loop" <- w56
  }
  n24 = node-c288(w1) -> ()  [unwired: 1 out]
  n25 = call "USB5CloseDevice.vi"("错误输入（无错误）"=w28, "DevIndex"=w27) -> ("error out"=→"error out":errorcluster)  [unwired: 8 in, 1 out]
